vi "Get Syntax In Global.vi"(8 "error in":errorcluster, 11 "System no.":i32) -> (0 "error out":errorcluster, 2 "Syntax":T1)   [LabVIEW 2020]
uses:
  Syntax.ctl
  Global1.vi
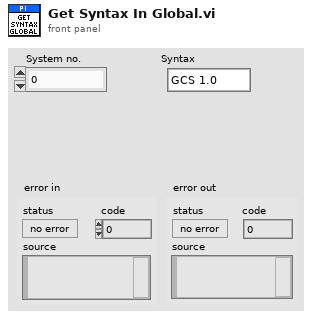
[diagram p1: front panel]
types:
  T1 = typedef "Syntax.ctl" = enum16{"GCS 1.0", "GCS 2.0", "GCS 3.0"}
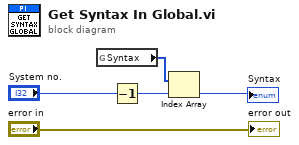
[diagram p0: block diagram]
diagram:
  n1 = global read "Global1.vi" "Syntax"() -> (w1:T1[])
  n2 = Decrement(x="System no.") -> (x-1=w2:i32)
  n3 = Index Array(array=w1, index=w2) -> (element=→"Syntax":T1)
  "error out" <- "error in"
